vi "subGeneratePackets (Bitstream).vi"(0 "PN sequence order\nfor Sync Bits":i32, 1 "PSK system parameters":T2, 2 "Packet Pad \n[samples]":i32, 5 "message bitstream":i8[](array[numeric]), 7 "Packet Parameters":T1, 9 "Message Type":bool, 12 "Samples per Symbol":i32, 13 "Tx IQ Sampling\nRate [s/sec]":dbl, 14 "Pulse Shaping Filter Parameters":T3) -> (4 "Packets":cluster{"t0":dbl, "dt":dbl, "Y":cdb[]}[](array[cluster]), 6 "Symbol Rate":dbl, 8 "Number of Packets":i32)   [LabVIEW 2013]
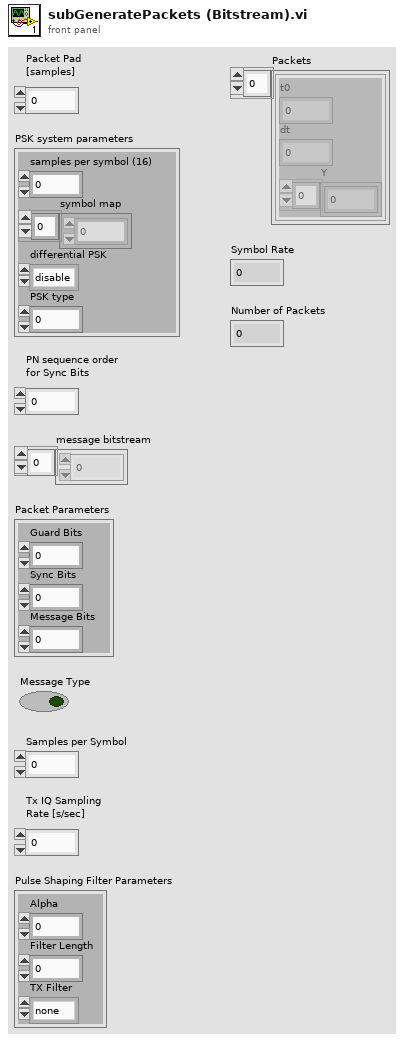
[diagram p1: front panel]
types:
  T1 = cluster{"Guard Bits ":i32, "Sync Bits":i32, "Message Bits":i32}
  T2 = cluster{"samples per symbol (16)":i32, "symbol map":cdb[], "differential PSK":enum16{"disable", "enable"}, "PSK type":u16}
  T3 = cluster{"Alpha":dbl, "Filter Length":i32, "TX Filter":enum16{"none", "Raised Cosine", "Root Raised Cos", "Gaussian"}}
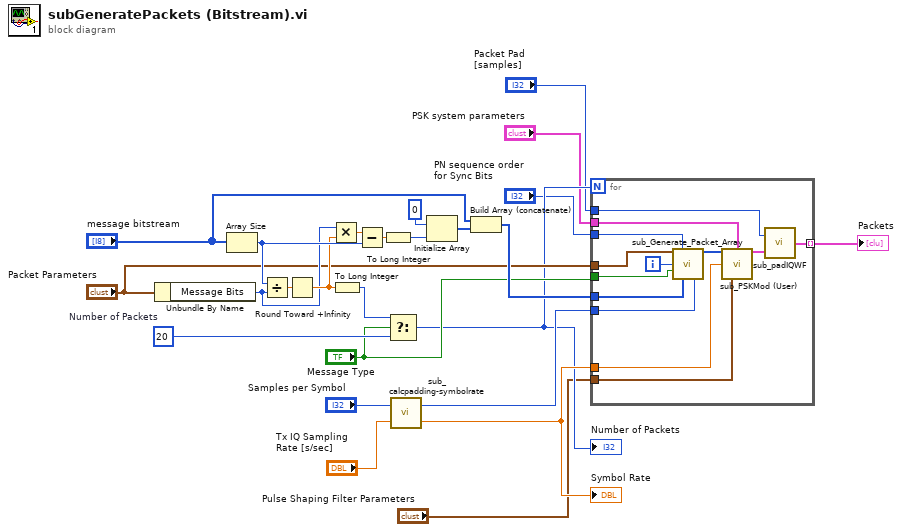
[diagram p0: block diagram]
diagram:
  w7 = 20  # Number of Packets
  n1 = Unbundle By Name("Packet Parameters") -> ("Message Bits"=w16:i32)
  n2 = Array Size(array="message bitstream") -> (size(s)=w19:i32)
  n3 = Divide(x=w19, y=w16) -> (x/y=w14:dbl)
  n4 = Round Toward +Infinity(x=w14) -> (ceil(x): smallest int >= x=w17:dbl)
  n5 = Multiply(x=w16, y=w17) -> (x*y=w18:dbl)
  n6 = To Long Integer(number=w17) -> (32bit integer=w15:i32)
  n7 = Subtract(x=w18, y=w19) -> (x-y=w20:dbl)
  n8 = To Long Integer(number=w20) -> (32bit integer=w23:i32)
  n9 = Select(t=w15, s="Message Type", f=w7) -> (s? t:f=w5:i32)
  "Number of Packets" <- w5
  n10 = call "sub_calcpadding-symbolrate.vi"("Tx IQ Sampling\nRate [s/sec]"="Tx IQ Sampling\nRate [s/sec]", "Samples per Symbol"="Samples per Symbol") -> ("Symbol Rate"=w12:dbl, "Padding Bits"=w10:i32)
  "Symbol Rate" <- w12
  n11 = Initialize Array(i8 0 ("element"), w23) -> (w22:i8[])
  n12 = Build Array (concatenate)("message bitstream", w22) -> (w25:i8[])
  n13 = for {
    N: w5 -> [_]
    tunnel: "Packet Parameters" -> [w35]
    tunnel: [w32] -> w8 mode=indexing
    tunnel: "Message Type" -> [w37]
    tunnel: w25 -> [w36]
    tunnel: "PN sequence order\nfor Sync Bits" -> [w34]
    tunnel: w10 -> [w33]
    tunnel: "PSK system parameters" -> [w30]
    tunnel: w12 -> [w28]
    tunnel: "Pulse Shaping Filter Parameters" -> [w29]
    tunnel: "Packet Pad \n[samples]" -> [w31]
    i -> [w38]
    n14 = call "sub_Generate_Packet_Array.vi"("Packet Parameters"=w35, "PN sequence order\nfor Sync"=w34, "Packet Number"=w38, "User defined bitstream?"=w37, "user  bitstream"=w36, "Cyclic Padding Bits"=w33) -> ("Output Packet"=w27:i8[])  [unwired: 9 in]
    n15 = call "sub_PSKMod (User).vi"("Packet to Transmit"=w27, "PSK system parameters"=w30, "Symbol Rate, Hz"=w28, "filter parameters"=w29) -> ("output complex waveform"=w26:cluster{"t0":dbl, "dt":dbl, "Y":cdb[]})  [unwired: 9 in, 2 out]
    n16 = call "sub_padIQWF.vi"("input complex waveform"=w26, "Packet Pad \n[samples]"=w31) -> ("output complex waveform"=w32:cluster{"t0":dbl, "dt":dbl, "Y":cdb[]})
  }
  "Packets" <- w8
